vi "exersise 3-1.vi"() -> ()   [LabVIEW 2014]
panel:
  out "warning":bool
  out "warning text":string
  in  "Min Temp":dbl
  in  "Max Temp":dbl
  in  "Current Temp":dbl
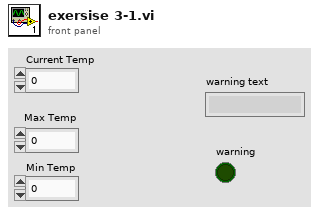
[diagram p1: front panel]
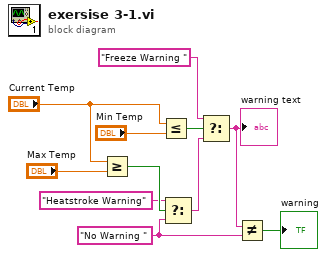
[diagram p0: block diagram]
diagram:
  w6 = "No Warning "
  n1 = Greater Or Equal?(x="Current Temp", y="Max Temp") -> (x >= y?=w8:bool)
  n2 = Less Or Equal?(x="Current Temp", y="Min Temp") -> (x <= y?=w7:bool)
  n3 = Select(t="Heatstroke Warning", s=w8, f=w6) -> (s? t:f=w4:string)
  n4 = Select(t="Freeze Warning ", s=w7, f=w4) -> (s? t:f=w2:string)
  "warning text" <- w2
  n5 = Not Equal?(x=w2, y=w6) -> (x != y?=→"warning":bool)
